vi "_Define connected systems (Array).vi"(0 "System no.":i32=1 min=1 max=4 step=1, 2 "Controller names":T1[](array[typedef]), 3 "Change only one system?":bool, 5 "error in":errorcluster) -> (19 "error out":errorcluster)   [LabVIEW 2012]
doc: "Defines connected systems and writes controller names into Global2 (Array).vi. This VI is called automatically by \"XXXX_Configuration_Setup.vi\" (with XXXX being the PI product number of your system) and must be completed successfully before\"General wait for movement to stop.vi\" is called. If \"Change only one system?\" is FALSE, all entries from \"Controller names\" are written into Global2 (Array).vi. If \"Change only one system?\" is TRUE, only the first field of \"Controller names\" is valid and only the entry for the given system number is overwritten in Global2 (Array).vi.\n\nValid for all systems.\n\nAnalog system: Only supported when called by Analog_Configuration_Setup.vi"
uses:
  mystage.llb/Controller names.ctl
  mystage.llb/Global2 (Array).vi
panel:
  # "Defines connected systems and writes controller names into Global2 \n(Array).vi. If \"Change only one system?\" is FALSE, all entries from \n\"Controller names\" are written into Global2 (Array).vi. If \"Change only \none system?\" is TRUE, only the first field of \"Controller names\" is valid \nand only the entry for the given system number is overwritten in \nGlobal2 (Array).vi."
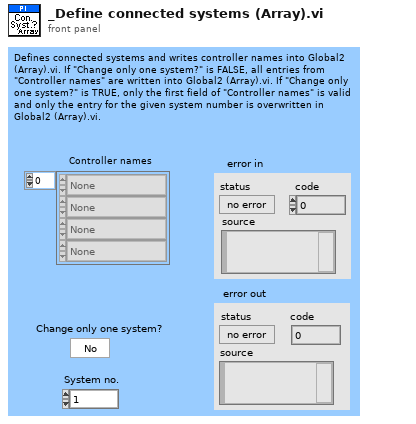
[diagram p1: front panel]
types:
  T1 = typedef "Controller names.ctl" = enum16{"None", "Analog", "C-702", "C-843", "C-843.PM", "C-844", "C-848", "C-865", "C-866", "C-867", "C-880", "E-516", "E-517", "E-710", "E-712", "E-725", "E-753", "E-755", "E-761", "E-816", "E-861", "F-206", "M-840", "M-850", "M-8X0", "Mercury"}
  T2 = cluster{"Conn. axes":string[], "Controller name":T1}[]
  T3 = cluster{"Conn. axes":string[], "Controller name":T1}
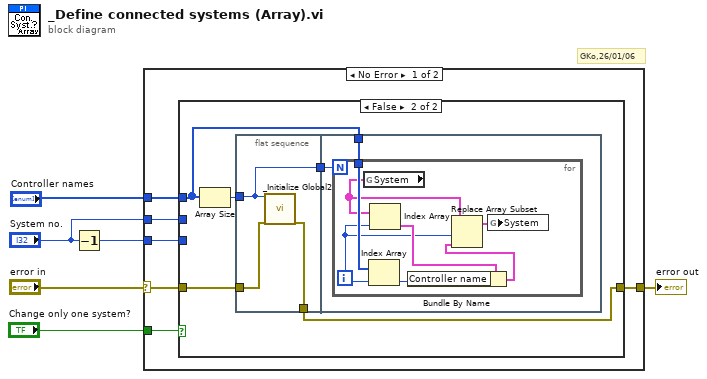
[diagram p0: block diagram]
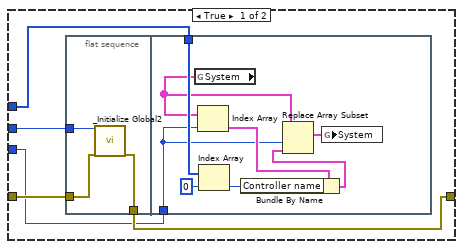
[diagram p2: hidden frame]
diagram:
  # "GKo,26/01/06"
  n1 = Decrement(x="System no.") -> (x-1=w3:i32)
  n2 = case shown="No Error" "error in" {
    selector: "error in" -> [w7 w46]
    tunnel: "Controller names" -> [w12 _]
    tunnel: [w10 w46] -> w6
    tunnel: "Change only one system?" -> [w11 _]
    tunnel: w3 -> [w9 _]
    tunnel: "System no." -> [w8 _]
    frame No Error {
      n3 = case shown="False" w11 {
        tunnel: w12 -> [w14 w31]
        tunnel: w7 -> [w16 w33]
        tunnel: [w15 w32] -> w10
        tunnel: w9 -> [w13 _]
        tunnel: w8 -> [w17 _]
        frame True {
          n4 = flat-sequence {
            tunnel: w17 -> [w20]
            tunnel: w16 -> [w19]
            tunnel: [w18] -> w15
            tunnel: w14 -> [w28]
            tunnel: w13 -> [w23]
            frame #0 {
              n5 = call "_Initialize Global2.vi"("System no."=w20, "error in"=w19) -> ("error out"=w18:errorcluster)  [unwired: 17 in]
            }
            frame #1 {
              n6 = global read "Global2 (Array).vi" "System"() -> (w27:T2)
              n7 = Index Array(array=w27, index=w23) -> (element=w26:T3)
              n8 = Index Array(array=w28, index=0) -> (element=w25:T1)
              n9 = Bundle By Name(cluster=w26, "Controller name"=w25) -> (w24:T3)
              n10 = Replace Array Subset(array=w27, new element=w24, index=w23) -> (w22:T2)
              n11 = global write "Global2 (Array).vi" "System"(w22) -> ()
            }
          }
        }
        frame False {
          n12 = Array Size(array=w31) -> (size(s)=w30:i32)
          n13 = flat-sequence {
            tunnel: w33 -> [w36]
            tunnel: [w35] -> w32
            tunnel: w30 -> [w34]
            tunnel: [w34] -> w29
            tunnel: w31 -> [w38]
            tunnel: w29 -> [w37]
            frame #0 {
              n14 = call "_Initialize Global2.vi"("System no."=w34, "error in"=w36) -> ("error out"=w35:errorcluster)  [unwired: 17 in]
            }
            frame #1 {
              n15 = for {
                N: w37 -> [_]
                tunnel: w38 -> [w45]
                i -> [w39]
                n16 = global read "Global2 (Array).vi" "System"() -> (w44:T2)
                n17 = Index Array(array=w45, index=w39) -> (element=w42:T1)
                n18 = Index Array(array=w44, index=w39) -> (element=w43:T3)
                n19 = Bundle By Name(cluster=w43, "Controller name"=w42) -> (w41:T3)
                n20 = Replace Array Subset(array=w44, new element=w41, index=w39) -> (w40:T2)
                n21 = global write "Global2 (Array).vi" "System"(w40) -> ()
              }
            }
          }
        }
      }
    }
    frame Error {
    }
  }
  "error out" <- w6
